vi "VPA QC File IO.vi"(10 "State Cluster In":T1, 11 "Function":enum16{"Read", "Write"}(ring)) -> (2 "State Cluster Out":T1)   [LabVIEW 2013]
uses:
  Controls/VPA QC State Data Cluster.ctl
  Controls/VPA QC General Cluster.ctl
  Controls/VPA QC State Enum.ctl
  Controls/VPA QC Bool Cluster.ctl
panel:
  # "Assembly Checklist"
  # "Assembly Checklist"
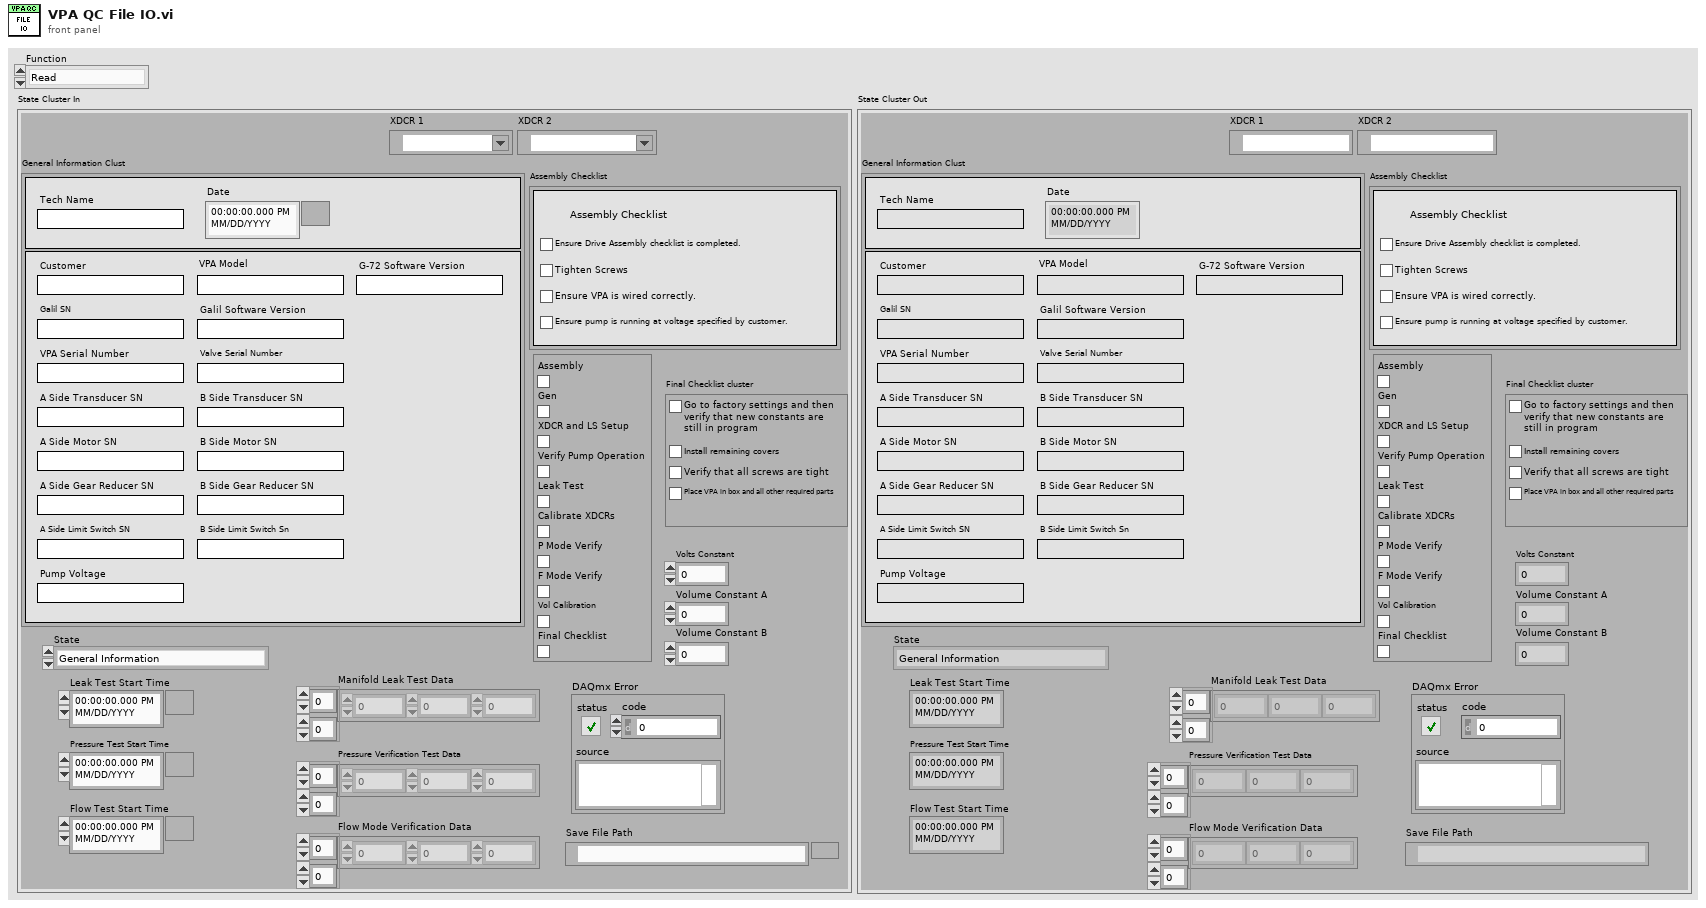
[diagram p1: front panel]
types:
  T1 = typedef "VPA QC State Data Cluster.ctl" = cluster{"XDCR 1":tag, "XDCR 2":tag, "General Information Clust":T2, "Assembly Checklist":cluster{"Ensure Drive Assembly checklist is completed.":bool, "Tighten Screws":bool, "Ensure VPA is wired correctly.":bool, "Ensure pump is running at voltage specified by customer.":bool}, "State":T3, "Manifold Leak Test Data":dbl[][], "Pressure Verification Test Data":dbl[][], "Flow Mode Verification Data":dbl[][], "DAQmx Error":errorcluster, "Bool Cluster":T4, "Leak Test Start Time":timestamp, "Pressure Test Start Time":timestamp, "Flow Test Start Time":timestamp, "Final Checklist cluster":cluster{"Check Fact Rest":bool, "Covers":bool, "Screws":bool, "Box":bool}, "Volts Constant":dbl, "Volume Constant A":dbl, "Volume Constant B":dbl, "Save File Path":path}
  T2 = typedef "VPA QC General Cluster.ctl" = cluster{"Tech Name":string, "Customer":string, "VPA Model":string, "G-72 Software Version":string, "Galil SN":string, "Galil Software Version":string, "VPA Serial Number":string, "Valve Serial Number":string, "A Side Transducer SN":string, "B Side Transducer SN":string, "A Side Motor SN":string, "B Side Motor SN":string, "A Side Gear Reducer SN":string, "B Side Gear Reducer SN":string, "A Side Limit Switch SN":string, "B Side Limit Switch Sn":string, "Pump Voltage":string, "Date":timestamp}
  T3 = typedef "VPA QC State Enum.ctl" = enum16{"General Information", "XDCR and LS Check", "Check Pump Function", "Manifold/Cylinder Leak Test", "Exit"}
  T4 = typedef "VPA QC Bool Cluster.ctl" = cluster{"Assembly":bool, "Gen":bool, "XDCR and LS Setup":bool, "Verify Pump Operation":bool, "Leak Test":bool, "Calibrate XDCRs":bool, "P Mode Verify":bool, "F Mode Verify":bool, "Vol Calibration":bool, "Final Checklist":bool}
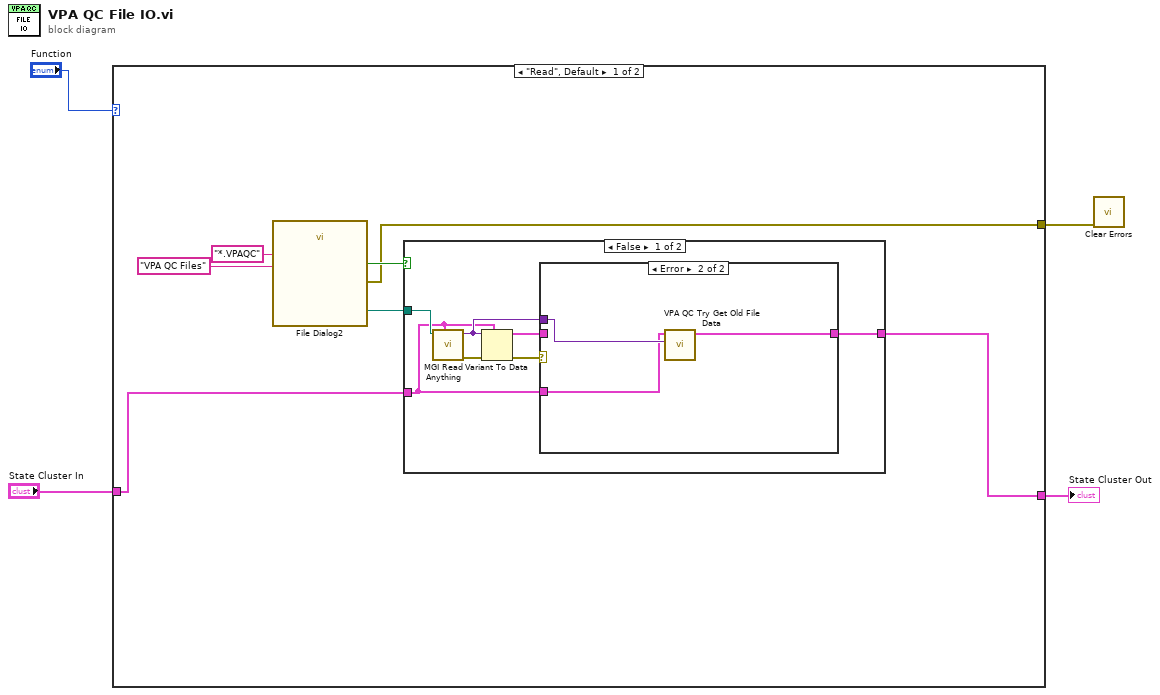
[diagram p0: block diagram]
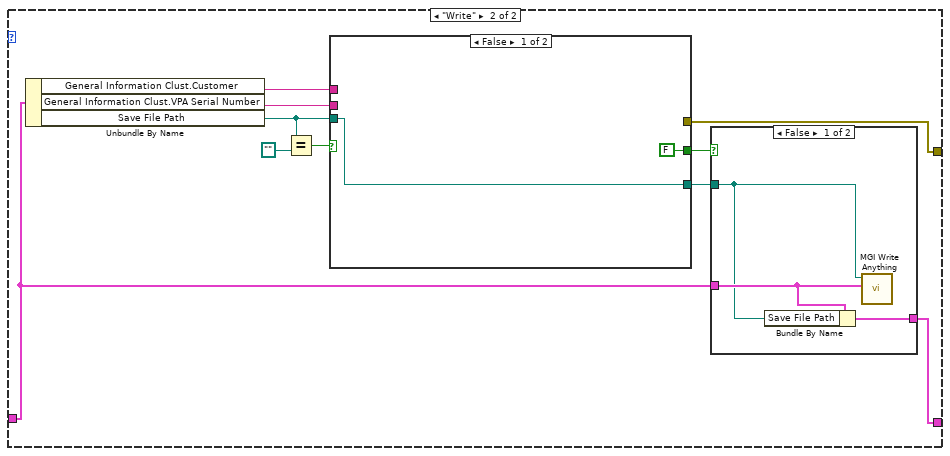
[diagram p4: hidden frame]
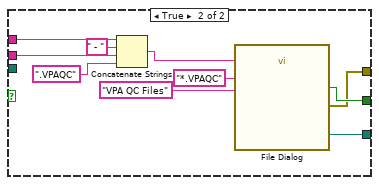
[diagram p5: hidden frame]
diagram:
  n1 = case shown="\"Read\", Default" "Function" {
    tunnel: "State Cluster In" -> [w8 w29]
    tunnel: [w6 w25] -> w2
    tunnel: [w5 w24] -> w1
    frame "Read", Default {
      n2 = call "File Dialog2"("pattern (all files)"="*.VPAQC", "pattern label"="VPA QC Files") -> ("selected path"=w9:path, "cancelled"=w7:bool, "error out"=w5:errorcluster)  [unwired: 10 in, 1 out]
      n3 = case shown="False" w7 {
        tunnel: w9 -> [w17 _]
        tunnel: w8 -> [w12 w23]
        tunnel: [w14 w23] -> w6
        frame False {
          n4 = call <userlib>:"MGI Read Anything.vi"("Type of Anything"=w12, "Path (dialog)"=w17) -> ("Error Out"=w18:errorcluster, "Anything"=w13:variant)  [unwired: 6 in, 2 out]
          n5 = Variant To Data(error in=w18, type=w12, Variant=w13) -> (data=w15:T1, error out=w16:errorcluster)
          n6 = case shown="Error" w16 {
            tunnel: w15 -> [w19 _]
            tunnel: [w19 w21] -> w14
            tunnel: w13 -> [_ w22]
            tunnel: w12 -> [_ w20]
            frame No Error {
            }
            frame Error {
              n7 = call "VPA QC Try Get Old File Data.vi"("File Data"=w22, "State Data In"=w20) -> ("State Cluster Out"=w21:T1)  [unwired: 9 in]
            }
          }
        }
        frame True {
        }
      }
    }
    frame "Write" {
      n8 = Unbundle By Name(w29) -> ("General Information Clust.Customer"=w33:string, "General Information Clust.VPA Serial Number"=w32:string, "Save File Path"=w26:path)
      n9 = Equal?(x=w26, y=path "") -> (x = y?=w27:bool)
      n10 = case shown="False" w27 {
        tunnel: w33 -> [_ w45]
        tunnel: w32 -> [_ w44]
        tunnel: [FALSE ("cancelled") w38] -> w31
        tunnel: [w35 w37] -> w30
        tunnel: w26 -> [w35 _]
        tunnel: [_ w36] -> w24
        frame False {
        }
        frame True {
          n11 = Concatenate Strings(w45, " - " ("string"), w44, ".VPAQC" ("string")) -> (w41:string)
          n12 = call "File Dialog"("default name"=w41, "pattern (all files)"="*.VPAQC", "pattern label"="VPA QC Files") -> ("selected path"=w37:path, "cancelled"=w38:bool, "error out"=w36:errorcluster)  [unwired: 9 in, 1 out]
        }
      }
      n13 = case shown="False" w31 {
        tunnel: w30 -> [w47 _]
        tunnel: w29 -> [w48 w49]
        tunnel: [w46 w49] -> w25
        frame False {
          n14 = Bundle By Name(cluster=w48, "Save File Path"=w47) -> (w46:T1)
          n15 = call <userlib>:"MGI Write Anything.vi"("Anything"=w48, "Path (dialog)"=w47) -> ()  [unwired: 7 in, 3 out]
        }
        frame True {
        }
      }
    }
  }
  "State Cluster Out" <- w2
  n16 = call <vilib>:"Clear Errors.vi"("error in (no error)"=w1) -> ()  [unwired: 6 in, 1 out]
